vi "SerialReadDHT11.vi"() -> ()   [LabVIEW 2017]
uses:
  <vilib>/Instr/_visa.llb/VISA Configure Serial Port (Instr).vi
panel:
  in  "Filename":path=path "C:/Users/AndrewCox/Documents/Labview_sketches/SerialReadDHT11/Testing1.xlsx"
  out "Humidity Chart":dbl[](graph)
  out "Humidity Gauge":dbl(knob) scale=0.0..100.0
  out "Saving Data":bool
  out "Filename Out":path
  in  "Enable":bool=TRUE
  out "Serial Data RAW":i32 format="%_3f"
  in  "Boolean":bool
  in  "baud rate (9600)":u32=9600
  in  "STOP DAQ":bool
  in  "VISA resource name":refnum<visa-resource-name>
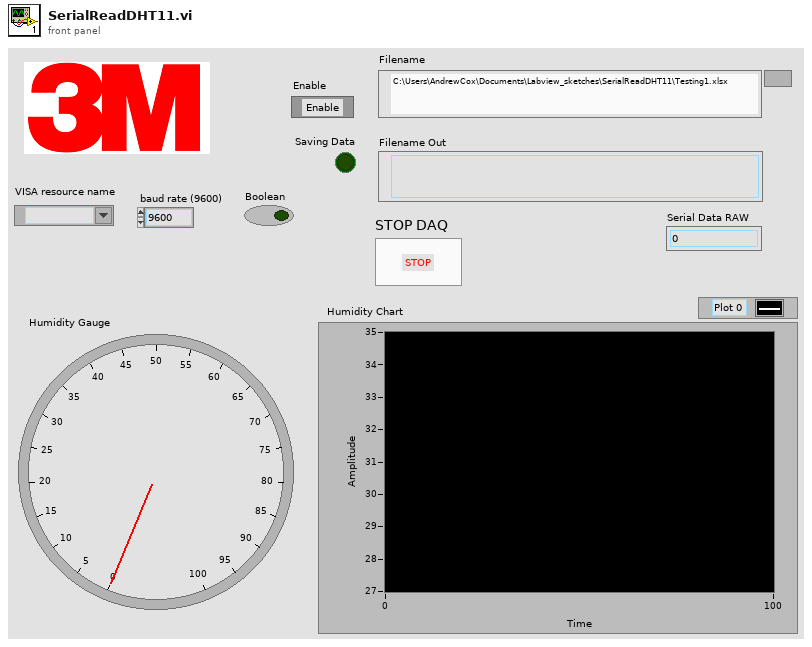
[diagram p1: front panel]
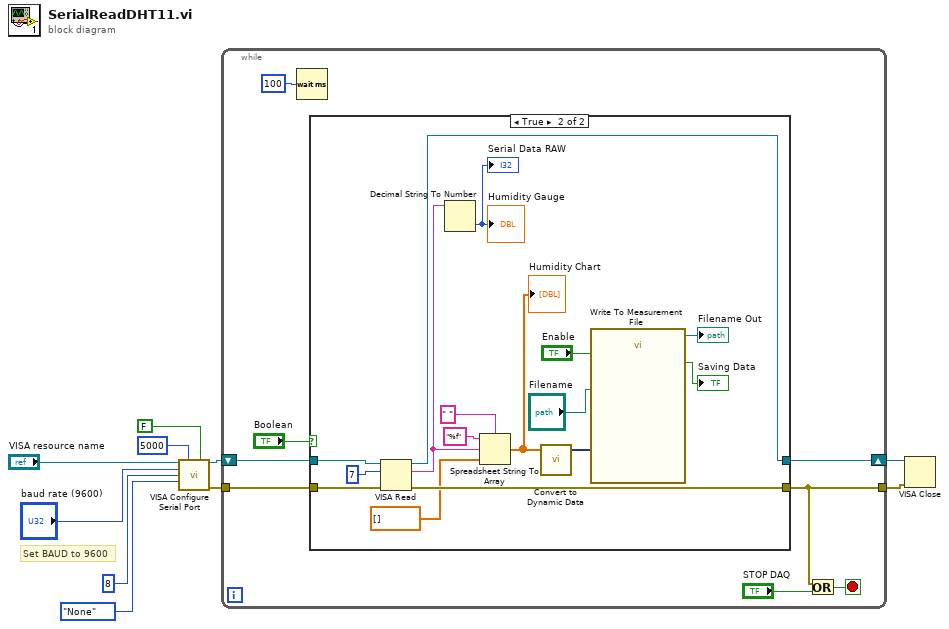
[diagram p0: block diagram]
diagram:
  # "Set BAUD to 9600"
  n1 = call-poly "VISA Configure Serial Port"("VISA resource name"="VISA resource name", "timeout (10sec)"=u32 5000, "Enable Termination\nChar (T)"=FALSE ("Enable Termination\nChar (T)"), "baud rate (9600)"="baud rate (9600)", "data bits (8)"=u16 8, "parity (0:none)"=enum16{"None", "Odd", "Even", "Mark", "Space"}."None") -> ("VISA resource name out"=w4:refnum<visa-resource-name>, "error out"=w5:errorcluster)  [unwired: 3 in, 5 out]
  n2 = while {
    tunnel: w5 -> [w17]
    tunnel: [w14] -> w2
    shift-right: [w13] -> w1
    shift-left: w4 -> [w12]
    stop <- w15 stop-if-true
    n3 = Wait (ms)(milliseconds to wait=u32 100) -> ()  [unwired: 1 out]
    n4 = case shown="True" "Boolean" {
      tunnel: w12 -> [w20 w36]
      tunnel: w17 -> [w19 w35]
      tunnel: [w19 w34] -> w14
      tunnel: [w20 w30] -> w13
      frame False {
      }
      frame True {
        n5 = VISA Read(VISA resource name=w36, byte count=u32 7, error in (no error)=w35) -> (VISA resource name out=w30:refnum<visa-resource-name>, read buffer=w25:string, error out=w34:errorcluster)  [unwired: 1 out]
        n6 = Decimal String To Number(string=w25) -> (number=→"Serial Data RAW" →"Humidity Gauge":i32)  [unwired: 2 in, 1 out]
        n7 = Spreadsheet String To Array(delimiter (Tab)=" ", format string="%f", spreadsheet string=w25, array type (2D Dbl)=dbl[] []) -> (array=w22:dbl[])
        "Humidity Chart" <- w22
        n8 = call "Convert to Dynamic Data"("Array"=w22) -> ("Dynamic Data Type"=w29:dynamicdata)  [unwired: 3 in]
        n9 = call "Write To Measurement File"("Signals"=w29, "Enable"="Enable", "Filename"="Filename") -> ("Filename Out"=→"Filename Out":path, "Saving Data"=→"Saving Data":bool)  [unwired: 14 in, 1 out]
      }
    }
    n10 = Or(x=w14, y="STOP DAQ") -> (x .or. y?=w15:bool)
  }
  n11 = VISA Close(VISA resource name=w1, error in (no error)=w2) -> ()  [unwired: 1 out]
